vi "Delete user event.vi"(8 "error in (no error)":errorcluster, 11 "Measurement in":refnum<class "Measurement.lvclass">) -> (0 "error out":errorcluster, 3 "Measurement out":refnum<class "Measurement.lvclass">)   [LabVIEW 2020, in "Measurement.lvlib" / "Measurement.lvclass"]
uses:
  Measurement.lvclass
  Measurement.lvclass/Measurement.ctl
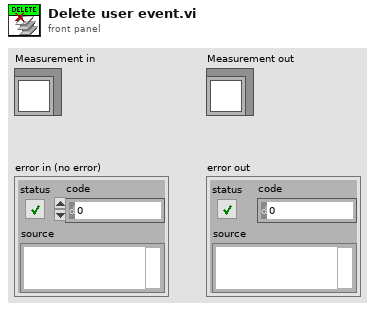
[diagram p1: front panel]
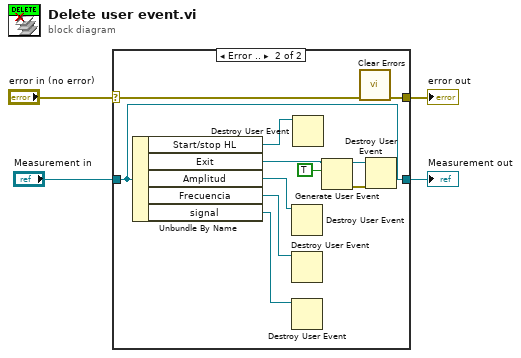
[diagram p0: block diagram]
diagram:
  n1 = case shown="Error .." "error in (no error)" {
    selector: "error in (no error)" -> [w5 w13]
    tunnel: "Measurement in" -> [w6 w11]
    tunnel: [w6 w11] -> w3
    tunnel: [w5 w12] -> w4
    frame No Error {
    }
    frame Error {
      n2 = Unbundle By Name(w11) -> ("Start/stop HL"=w17:refnum<user-event>, "Exit"=w9:refnum<user-event>, "Amplitud"=w16:refnum<user-event>, "Frecuencia"=w15:refnum<user-event>, "signal"=w14:refnum<user-event>)
      n3 = Destroy User Event(user event=w16) -> ()  [unwired: 1 in, 1 out]
      n4 = Destroy User Event(user event=w15) -> ()  [unwired: 1 in, 1 out]
      n5 = Destroy User Event(user event=w14) -> ()  [unwired: 1 in, 1 out]
      n6 = Destroy User Event(user event=w17) -> ()  [unwired: 1 in, 1 out]
      n7 = Generate User Event(user event=w9, event data cluster=TRUE ("event data")) -> (user event out=w8:refnum<user-event>, error out=w10:errorcluster)  [unwired: 2 in]
      n8 = call <vilib>:"Clear Errors.vi"("error in (no error)"=w13) -> ("error out"=w12:errorcluster)  [unwired: 5 in, 1 out]
      n9 = Destroy User Event(user event=w8, error in=w10) -> ()  [unwired: 1 out]
    }
  }
  "error out" <- w4
  "Measurement out" <- w3
